vi "copyWebcamFileToPics.vi"(9 "WebcamINIpath":path, 11 "BasePathOfPics":path) -> (2 "copyTo":path)   [LabVIEW 2022 SP3]
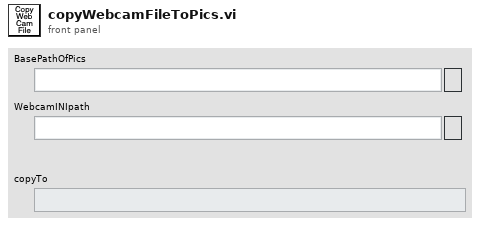
[diagram p1: front panel]
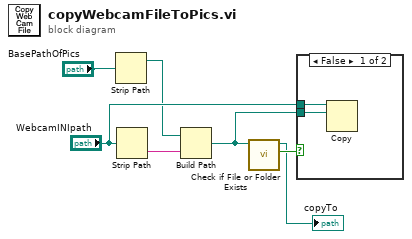
[diagram p0: block diagram]
diagram:
  n1 = Strip Path(path="BasePathOfPics") -> (stripped path=w5:path)  [unwired: 1 out]
  n2 = Strip Path(path="WebcamINIpath") -> (name=w4:string)  [unwired: 1 out]
  n3 = Build Path(base path=w5, name or relative path=w4) -> (appended path=w3:path)
  n4 = call <vilib>:"Check if File or Folder Exists.vi"("path"=w3) -> ("file or folder exists?"=w2:bool, "dup path"=→"copyTo":path)  [unwired: 8 in, 1 out]
  n5 = case shown="False" w2 {
    tunnel: "WebcamINIpath" -> [w9 _]
    tunnel: w3 -> [w8 _]
    frame False {
      n6 = Copy(10:w8, 11:w9) -> ()  [unwired: 3 in, 3 out]
    }
    frame True {
    }
  }
